vi "FRCts20_Backend_Team_GETIndex_reform.vi"(7 "Team":T1, 8 "error in (no error)":errorcluster, 11 "teamdata":variant[][](array[variant])) -> (0 "error out":errorcluster, 2 "data string":string)   [LabVIEW 2014, in "FRCts20_Backend_Engine.lvlib"]
doc: "Reforms and returns the specific team's data"
uses:
  FRCts20_Backend_Engine.lvlib
  FRCts20_Backend_API/FRCts20_Backend_API_Team.ctl
  FRCts20_Backend_API/FRCts20_Backend_API_SW.ctl
  FRCts20_Backend_API/FRCts20_Backend_API_Status.ctl
  <vilib>/addons/database/_DB Variant To Data/Database Variant To Data.xnode
  FRCts20_Backend_API/FRCts20_Backend_API.lvlib
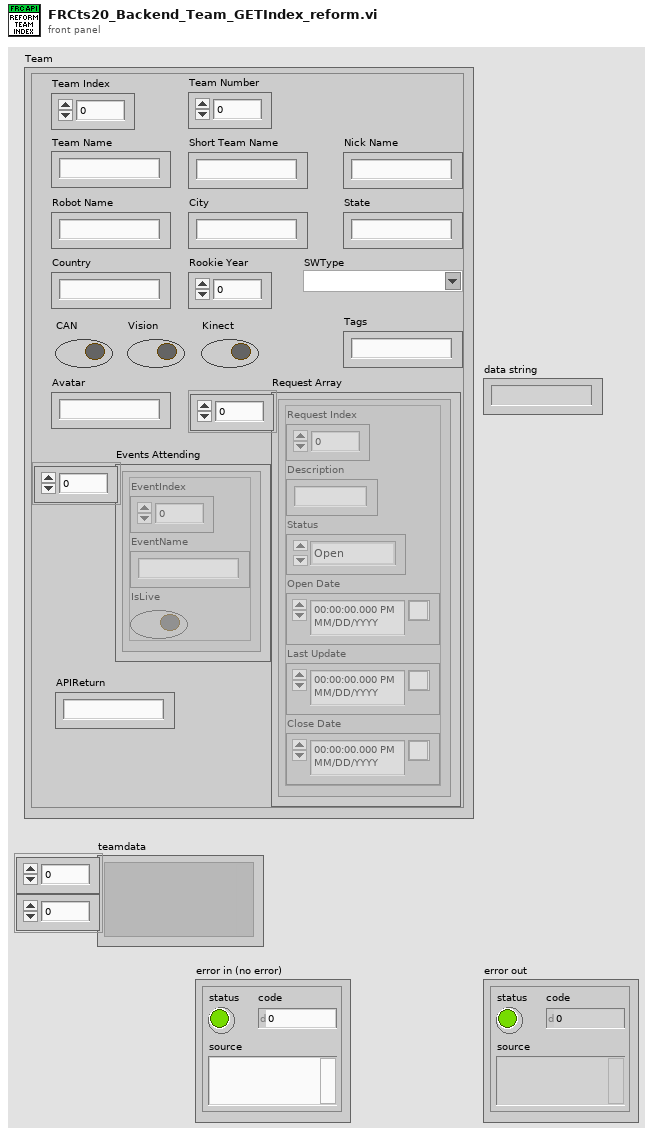
[diagram p1: front panel]
types:
  T1 = typedef "FRCts20_Backend_Engine.lvlib/FRCts20_Backend_API.lvlib/FRCts20_Backend_API_Team.ctl" = cluster{"Team Index":u32, "Team Number":u32, "Team Name":string, "Short Team Name":string, "Nick Name":string, "Robot Name":string, "City":string, "State":string, "Country":string, "Rookie Year":u32, "SWType":T2, "CAN":bool, "Vision":bool, "Kinect":bool, "Tags":string, "Avatar":string, "Request Array":cluster{"Request Index":u32, "Description":string, "Status":T3, "Open Date":timestamp, "Last Update":timestamp, "Close Date":timestamp}[], "Events Attending":cluster{"EventIndex":dbl, "EventName":string, "IsLive":bool}[], "APIReturn":string}
  T2 = typedef "FRCts20_Backend_Engine.lvlib/FRCts20_Backend_API.lvlib/FRCts20_Backend_API_SW.ctl" = string
  T3 = typedef "FRCts20_Backend_Engine.lvlib/FRCts20_Backend_API.lvlib/FRCts20_Backend_API_Status.ctl" = enum16{"Open", "In Work", "Closed"}
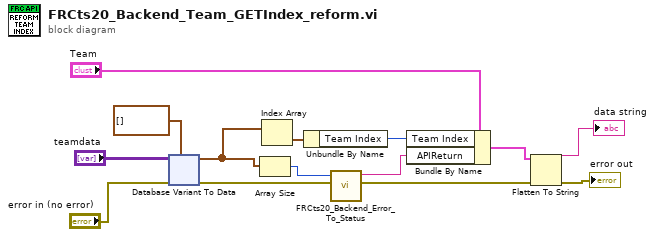
[diagram p0: block diagram]
diagram:
  n1 = xnode "Database Variant To Data"("database variant"="teamdata", "error in (no error)"="error in (no error)", "type"=cluster{"Team Index":u32}[] []) -> ("data"=w3:cluster{"Team Index":u32}[], "error out"=w8:errorcluster)
  n2 = Array Size(array=w3) -> (size(s)=w2:i32)
  n3 = Index Array(array=w3) -> (element=w7:cluster{"Team Index":u32})  [unwired: 1 in]
  n4 = Unbundle By Name(w7) -> ("Team Index"=w6:u32)
  n5 = call "FRCts20_Backend_Error_To_Status.vi"("error in (no error)"=w8, "rows affected"=w2) -> ("error out"=w13:errorcluster, "String"=w1:string)  [unwired: 8 in]
  n6 = Bundle By Name(cluster="Team", "Team Index"=w6, "APIReturn"=w1) -> (w4:T1)
  n7 = Flatten To String(anything=w4, error in (no error)=w13) -> (data string=→"data string":string, error out=→"error out":errorcluster)  [unwired: 2 in, 1 out]
